vi "robo_getIdn.vi"(0 "连接ID":refnum<k5>, 1 "错误输入（无错误）":errorcluster) -> (2 "连接ID输出":refnum<k5>, 3 "读取缓冲区":string, 4 "错误输出":errorcluster)   [LabVIEW 2017]
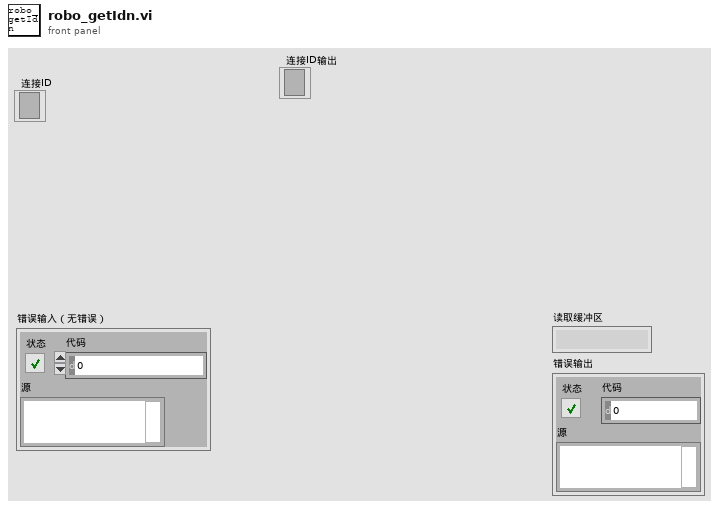
[diagram p1: front panel]
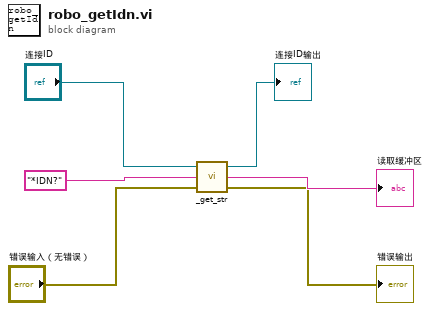
[diagram p0: block diagram]
diagram:
  n1 = call "_get_str.vi"("错误输入（无错误）"="错误输入（无错误）", "写入缓冲区"="*IDN?", "连接ID"="连接ID") -> ("错误输出"=→"错误输出":errorcluster, "读取缓冲区"=→"读取缓冲区":string, "连接ID输出"=→"连接ID输出":refnum<k5>)
